vi "Disconnect.vi"(8 "error in (no error)":errorcluster, 11 "Flash Utility in":refnum<class "Flash Utility.lvclass">) -> (0 "error out":errorcluster, 3 "Flash Utility out":refnum<class "Flash Utility.lvclass">)   [LabVIEW 2018, in "Flash Utility.lvlib" / "Flash Utility.lvclass"]
uses:
  Flash Utility.lvclass
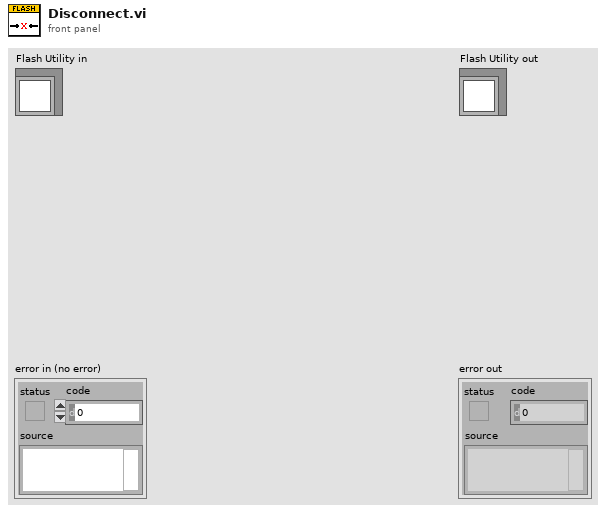
[diagram p1: front panel]
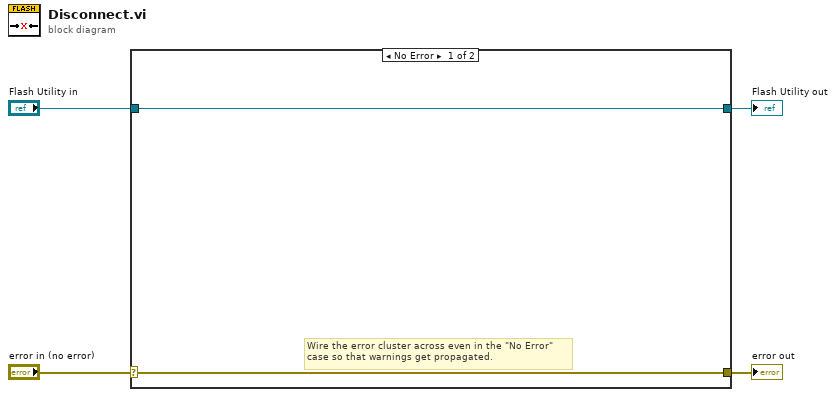
[diagram p0: block diagram]
diagram:
  n1 = case shown="No Error" "error in (no error)" {
    selector: "error in (no error)" -> [w5 w8]
    tunnel: [w5 w8] -> w3
    tunnel: [w6 w7] -> w1
    tunnel: "Flash Utility in" -> [w6 w7]
    frame No Error {
      # "Wire the error cluster across even in the \"No Error\"\ncase so that warnings get propagated."
    }
    frame Error {
    }
  }
  "error out" <- w3
  "Flash Utility out" <- w1
